vi "Write Current Power.vi"(8 "error in (no error)":errorcluster, 10 "Current Power":dbl, 11 "Laser State Data in":refnum<class "Laser State Data.lvclass">) -> (0 "error out":errorcluster, 3 "Laser State Data out":refnum<class "Laser State Data.lvclass">)   [LabVIEW 2022 SP3, in "Laser State Data.lvclass"]
uses:
  Laser State Data.lvclass
  Laser State Data.lvclass/Laser State Data.ctl
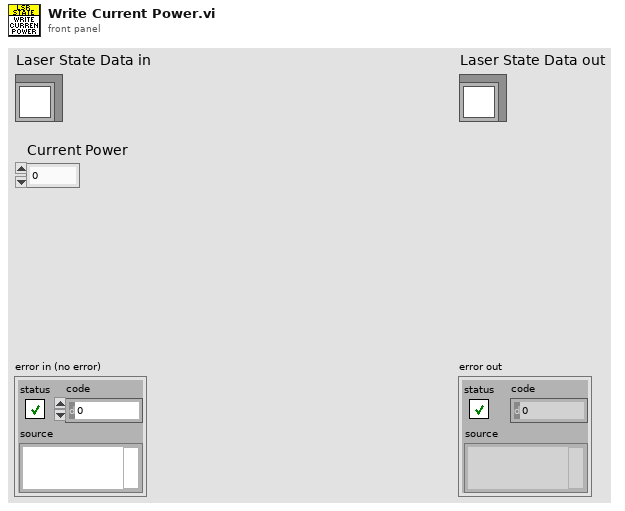
[diagram p1: front panel]
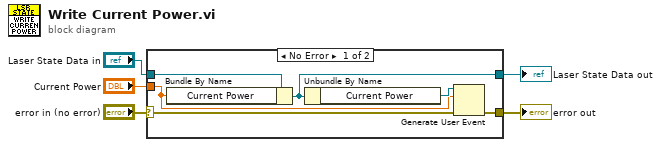
[diagram p0: block diagram]
diagram:
  n1 = case shown="No Error" "error in (no error)" {
    selector: "error in (no error)" -> [w7 w12]
    tunnel: [w6 w12] -> w4
    tunnel: [w10 w13] -> w2
    tunnel: "Laser State Data in" -> [w11 w13]
    tunnel: "Current Power" -> [w8 _]
    frame No Error {
      n2 = Bundle By Name(cluster=w11, "Current Power"=w8) -> (w10:refnum<class "Laser State Data.lvclass">)
      n3 = Unbundle By Name(w10) -> ("Current Power"=w9:refnum<user-event>)
      n4 = Generate User Event(user event=w9, event data cluster=w8, error in=w7) -> (error out=w6:errorcluster)  [unwired: 1 in, 1 out]
    }
    frame Error {
    }
  }
  "error out" <- w4
  "Laser State Data out" <- w2
